vi "somme_deux_signaux.vi"() -> ()   [LabVIEW 2018]
uses:
  <vilib>/express/express analysis/Spectral/Block/exnSpectralBlock spectral measurements power poly.vi
  <vilib>/express/express analysis/Spectral/Block/exnSpectralBlock spectral measurements power DDT.vi
  <vilib>/express/express analysis/Spectral/XNode/ExpressSpectralMeasurementsBlockNode.xnode
panel:
  out "Amplitude":dbl=1.0
  out "Frequency":dbl=0.05
  out "Waveform Graph 6":dynamicdata(graph)
  out "Waveform Graph 5":dynamicdata(graph)
  out "Waveform Graph 3":dynamicdata(graph)
  out "Waveform Graph":dynamicdata(graph)
  in  "stop":bool
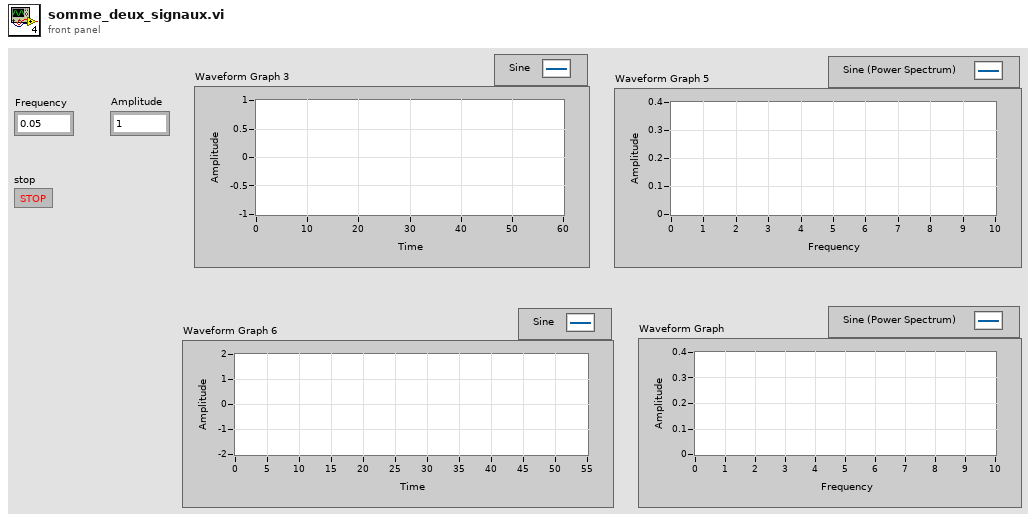
[diagram p1: front panel]
types:
  T1 = cluster{"averaging mode":u16, "weighting mode":u16, "number of averages":u32}
  T2 = cluster{"dB On (F)":bool, "unwrap phase (F)":bool, "convert to degree (F)":bool}
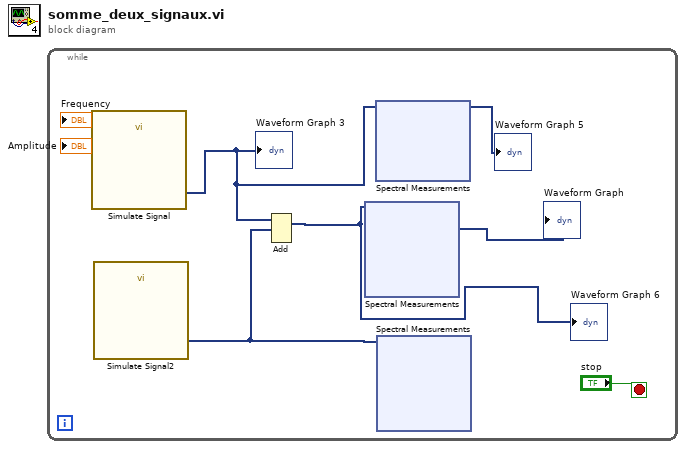
[diagram p0: block diagram]
diagram:
  n1 = while {
    stop <- "stop" stop-if-true
    n2 = call "Simulate Signal"() -> ("Sine"=w5:dynamicdata)  [unwired: 14 in, 1 out]
    "Waveform Graph 3" <- w5
    n3 = call "Simulate Signal2"() -> ("Sine"=w2:dynamicdata)  [unwired: 14 in, 1 out]
    n4 = Add(1:w2, 2:w5) -> (0:w1:dynamicdata)  [unwired: 1 in, 1 out]
    "Waveform Graph 6" <- w1
    n5 = xnode "Spectral Measurements"("Signals"=w1) -> ("Power Spectrum"=→"Waveform Graph":dynamicdata)  [unwired: 1 in, 1 out]
    n6 = xnode "Spectral Measurements"("Signals"=w5) -> ("Power Spectrum"=→"Waveform Graph 5":dynamicdata)  [unwired: 1 in, 1 out]
    n7 = xnode "Spectral Measurements"("Signals"=w2) -> ()  [unwired: 1 in, 2 out]
  }
